vi "crop_input_images.vi"() -> ()   [LabVIEW 2011]
uses:
  global_vars.vi
  <vilib>/Utility/file.llb/Write To Spreadsheet File (I64).vi
  <vilib>/vision/NI_Vision_Development_Module.lvlib
panel:
  in  "Numeric Control":dbl=0.454545454
  out "input_line_plot 2":dbl[][](graph)
  in  "Tab Control":T1(tab)
  out "input_line_plot":u8[][](graph)
  out "img_dist_input":T2(plugin-control)
  out "img_orig_input":T2(plugin-control)
  in  "i32_sel_input_image":i32
  in  "select row input":i32(slide) scale=0.0..1200.0
  in  "select row unwrapped":i32(slide) scale=0.0..1200.0
  out "img_dist_phaseMap":T2(plugin-control)
  out "img_orig_masked_with_dist":T2(plugin-control)
  out "noise_mask_line_plot":u8[](graph)
  out "img_noise_maks":T2(plugin-control)
  out "i32_First/last px":i32[][](graph)
  in  "select row":i32(slide) scale=0.0..1200.0
  out "last px":i32
  out "first px":i32
  in  "save data":bool
  out "i32_ar_displ_map":i32[][](array[numeric])
  in  "safety margin":i32=5
  out "u8_ar_noise_mask":u8[][](array[numeric])
  out "crunching numbers":bool
  out "Intensity Graph":i32[][](graph)
  out "u8_ar_orig_phase_masked_with_dist":u8[][](array[numeric])
  in  "noise threshold":dbl=20.0
  out "img_orig_unwrap":T2(plugin-control)
  in  "calc difference":bool
  out "Y Resolution":i32
  out "X Resolution":i32
  in  "update_cor":bool
  out "path_dist_files":path[](array[path])=[path "X:/Cloud Drives/Dropbox/Europhotonics/FringeMan/Image Storage/02_07/x-direction/dist/12_56_10-5.00fringes_0of4__capt_.png", path "X:/Cloud Drives/Dropbox/Europhotonics/FringeMan/Image Storage/02_07/x-direction/dist/12_56_10-5.00fringes_1of4__capt_.png", path "X:/Cloud Drives/Dropbox/Europhotonics/FringeMan/Image Storage/02_07/x-direction/dist/12_56_10-5.00fringes_2of4__capt_.png", path "X:/Cloud Drives/Dropbox/Europhotonics/FringeMan/Image Storage/02_07/x-direction/dist/12_56_10-5.00fringes_3of4__capt_.png"]
  out "path_orig_files":path[](array[path])=[path "X:/Cloud Drives/Dropbox/Europhotonics/FringeMan/Image Storage/02_07/x-direction/orig/12_56_10-5.00fringes_0of4__original_.png", path "X:/Cloud Drives/Dropbox/Europhotonics/FringeMan/Image Storage/02_07/x-direction/orig/12_56_10-5.00fringes_1of4__original_.png", path "X:/Cloud Drives/Dropbox/Europhotonics/FringeMan/Image Storage/02_07/x-direction/orig/12_56_10-5.00fringes_2of4__original_.png", path "X:/Cloud Drives/Dropbox/Europhotonics/FringeMan/Image Storage/02_07/x-direction/orig/12_56_10-5.00fringes_3of4__original_.png"]
  in  "dbl_ar_crop_correction":dbl[](array[numeric])=[0.0, 0.0, 0.0, 0.0] caption="crop_correction"
  in  "u8_y_center_cor":i16
  in  "u8_x_center_cor":i16=-20
  in  "radius correction":i16=-30
  out "img_dist_unwrap":T2(plugin-control)
  out "u8_ar_orig_phasemap":u8[][](array[numeric])
  out "dbl_pxar_orig_unwrap":u8[][](array[numeric])
  out "dbl_pxar_dist_unwrap":u8[][](array[numeric])
  out "u8_pxar_orig":u8[][][](array[numeric])
  in  "read orig":bool
  in  "read dist":bool
  out "u8_ar_dist_phasemap":u8[][](array[numeric])
  in  "calculate \nphase map":bool
  out "u8_pxar_dist":u8[][][](array[numeric])
  in  "Stop Button":bool
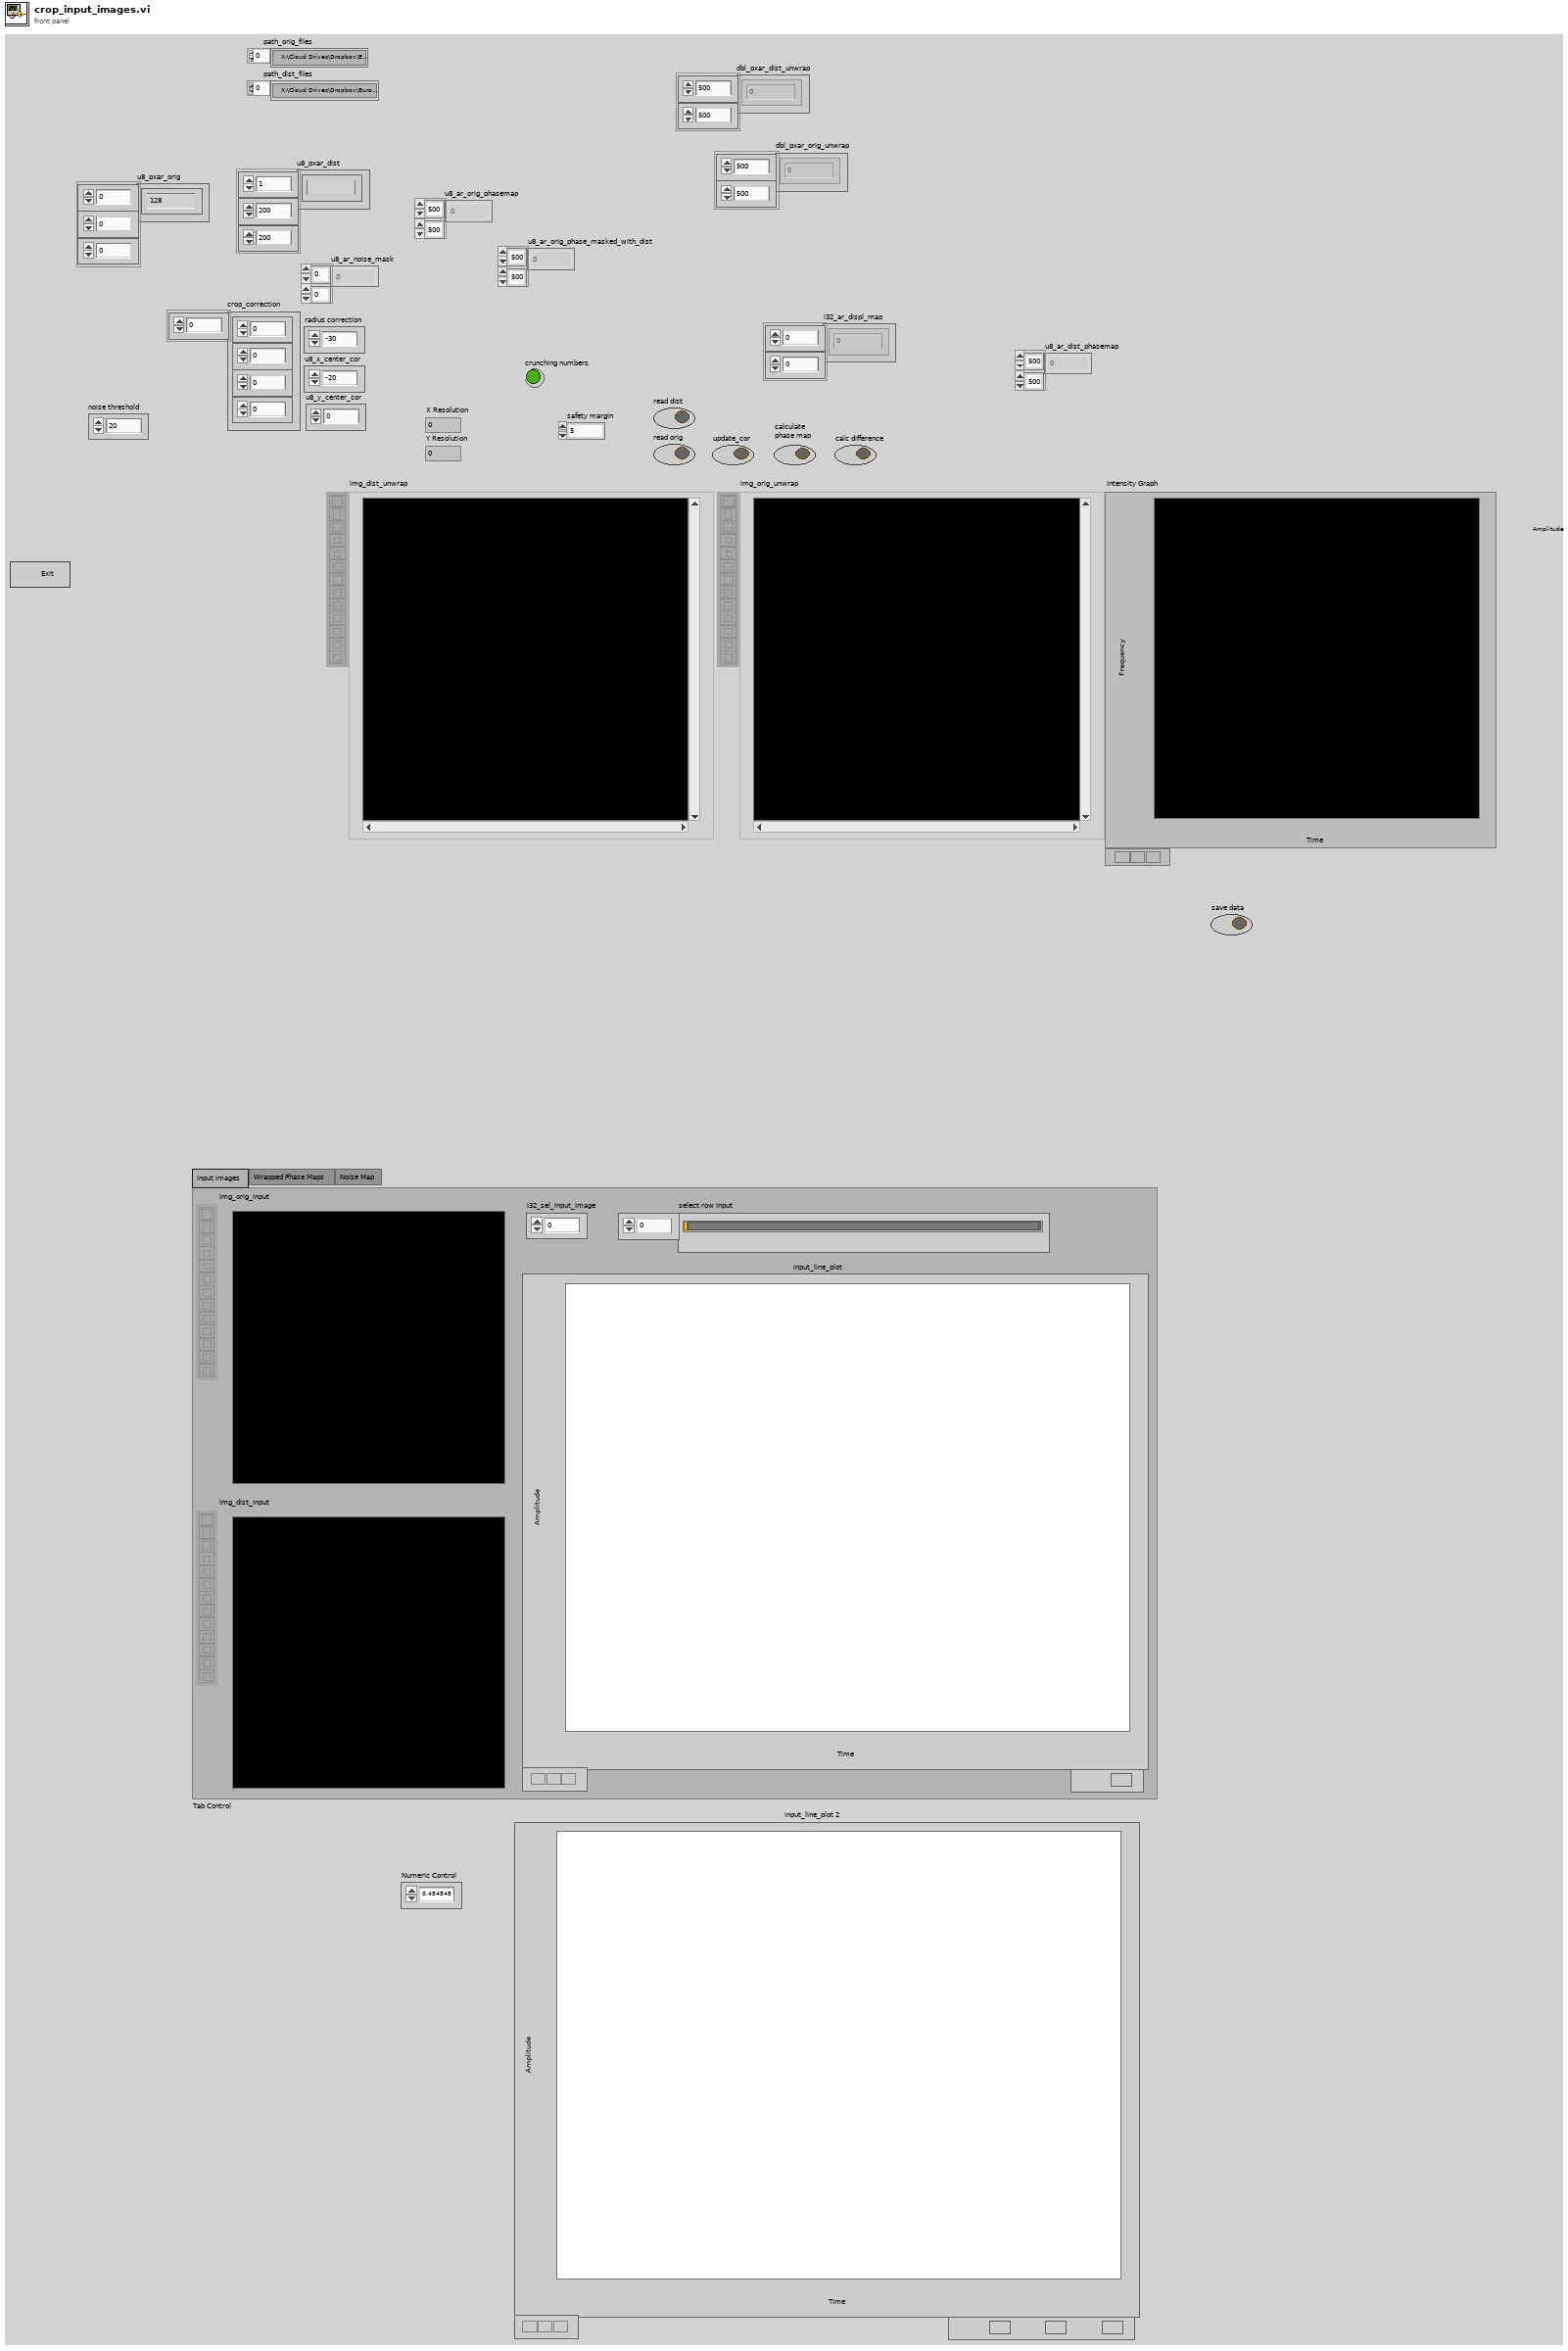
[diagram p1: front panel]
types:
  T1 = enum32{"Input Images", "Wrapped Phase Maps", "Noise Map"}
  T2 = typedef "IMAQ Image.ctl" = refnum<image>
  T3 = typedef "Image Type" = u32
  T4 = cluster{"radius correction":i16, "u8_x_center_cor":i16, "u8_y_center_cor":i16}
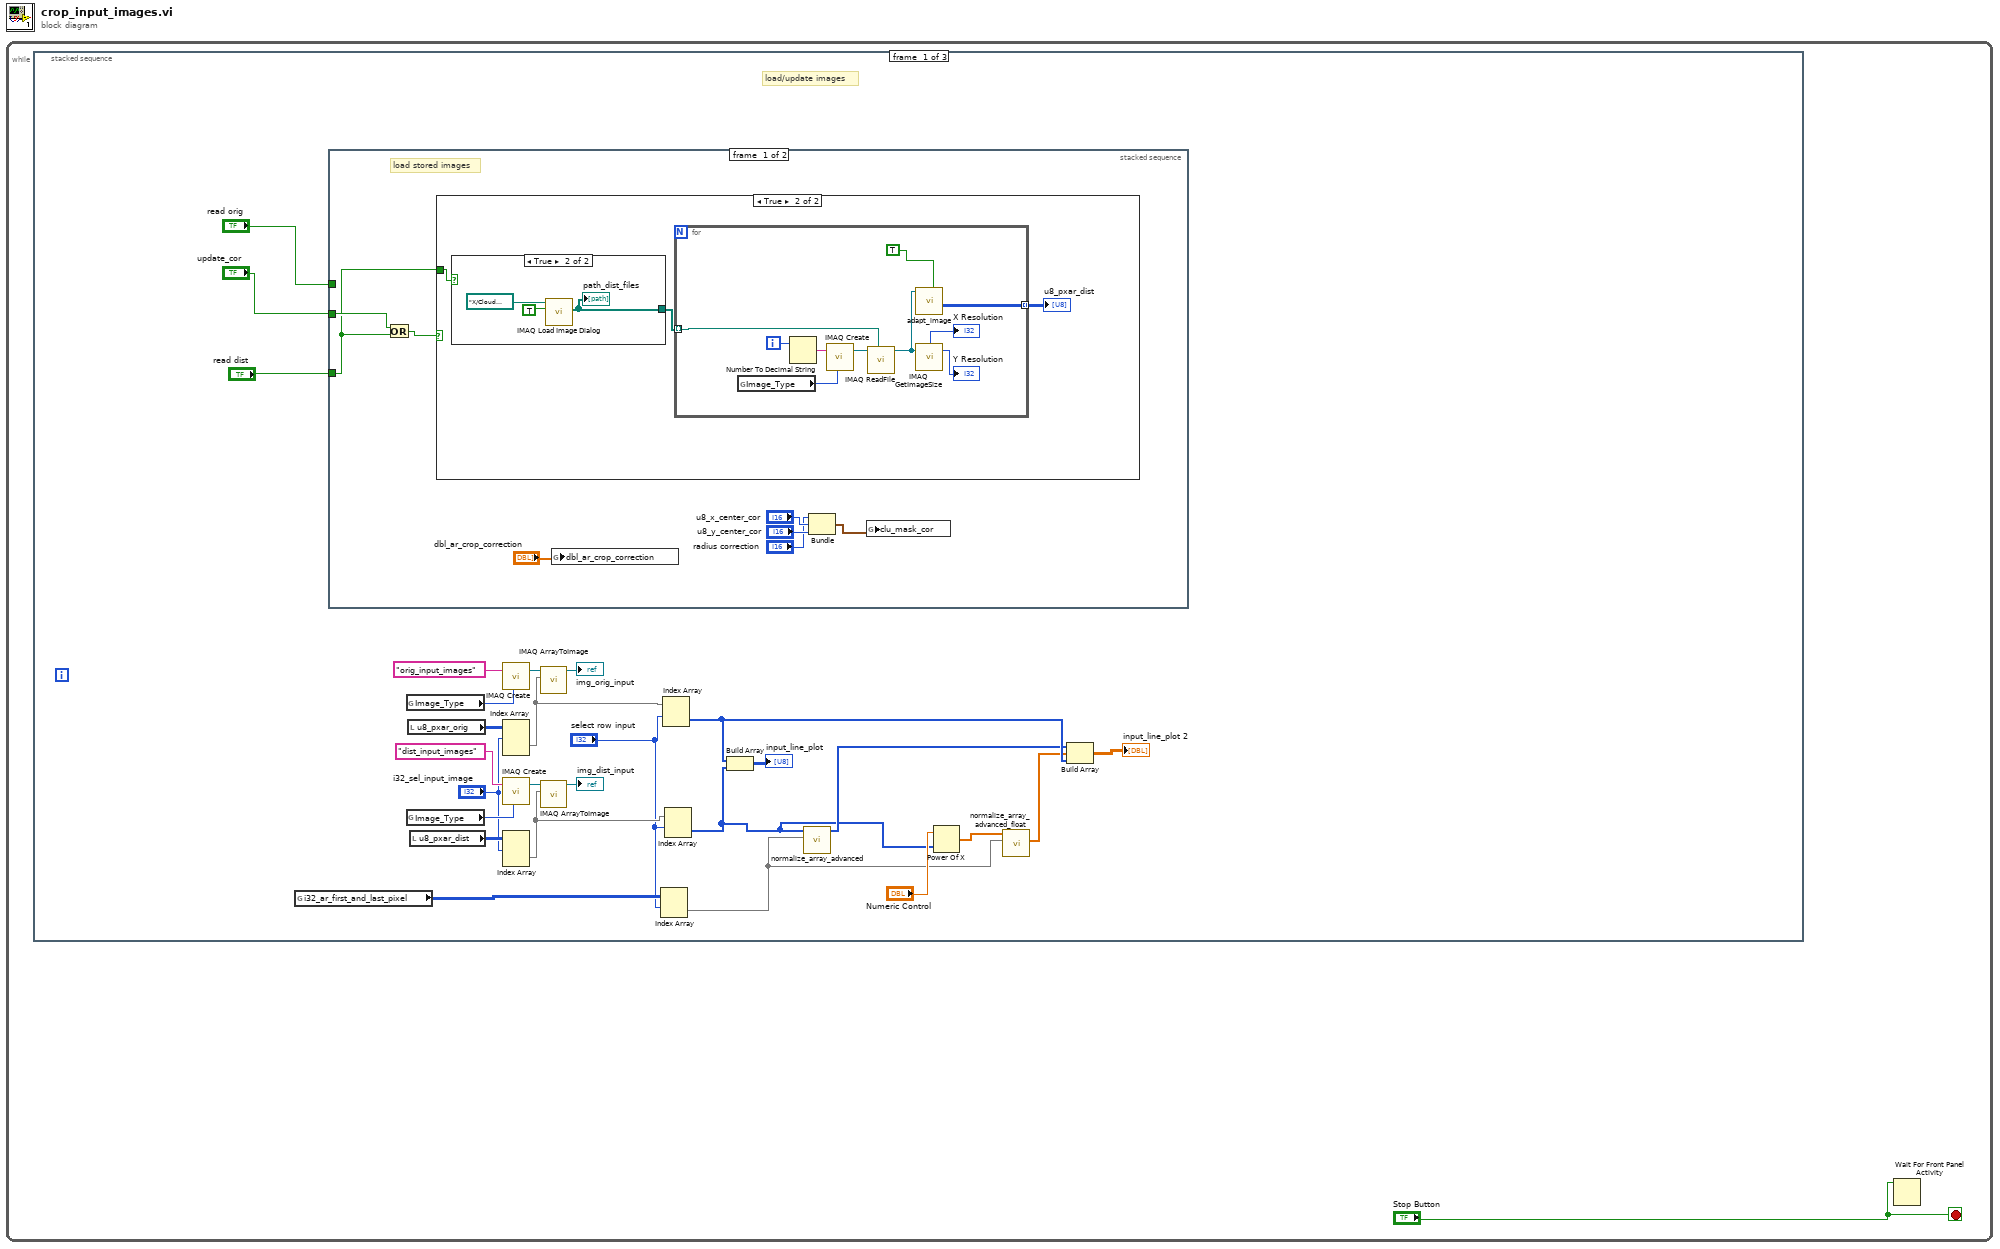
[diagram p0: block diagram]
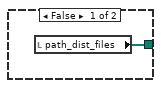
[diagram p3: hidden frame]
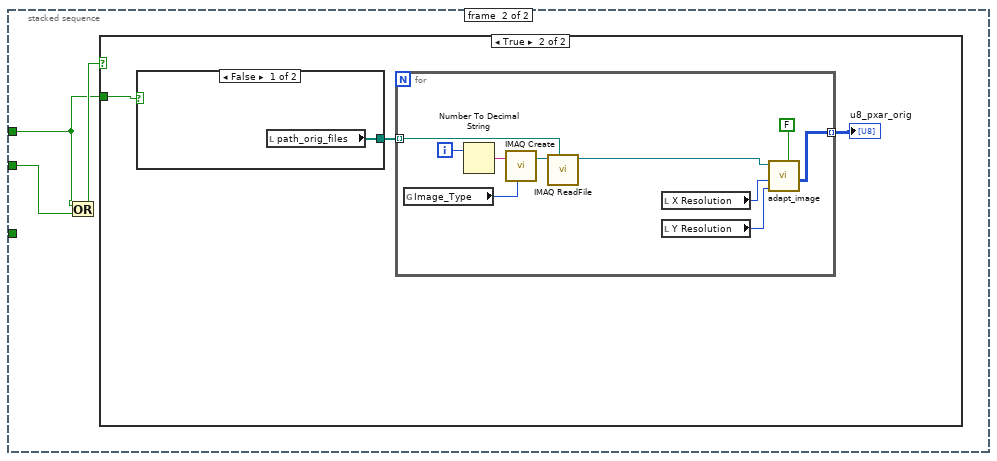
[diagram p4: hidden frame]
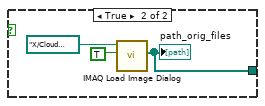
[diagram p6: hidden frame]
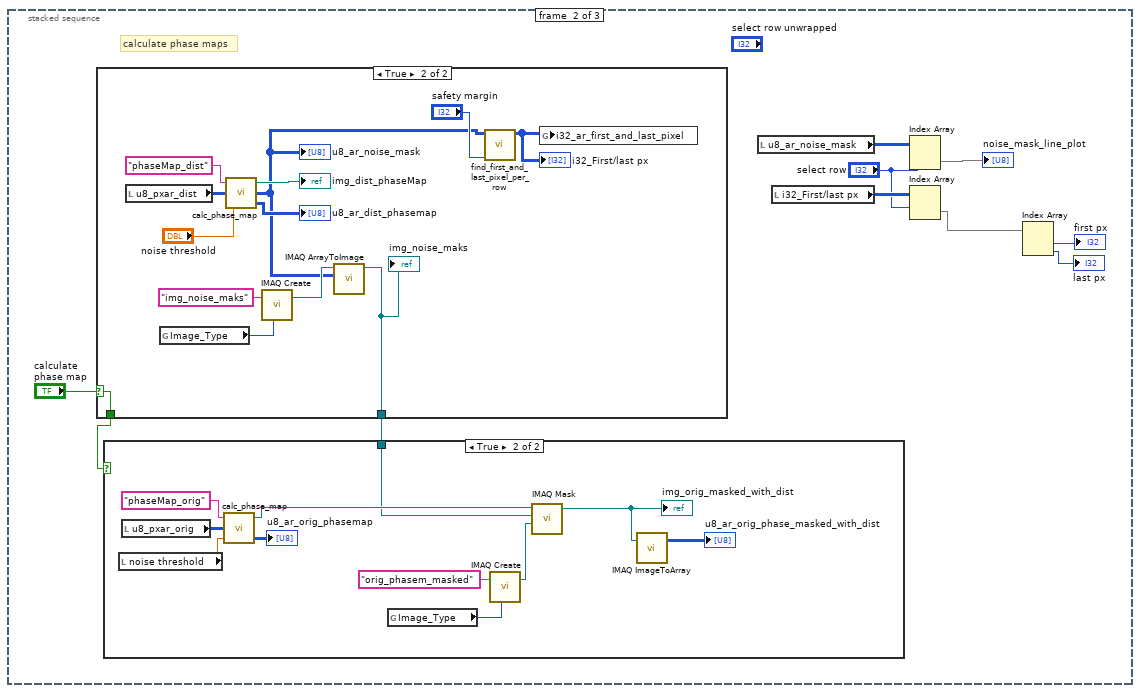
[diagram p7: hidden frame]
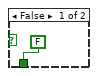
[diagram p9: hidden frame]
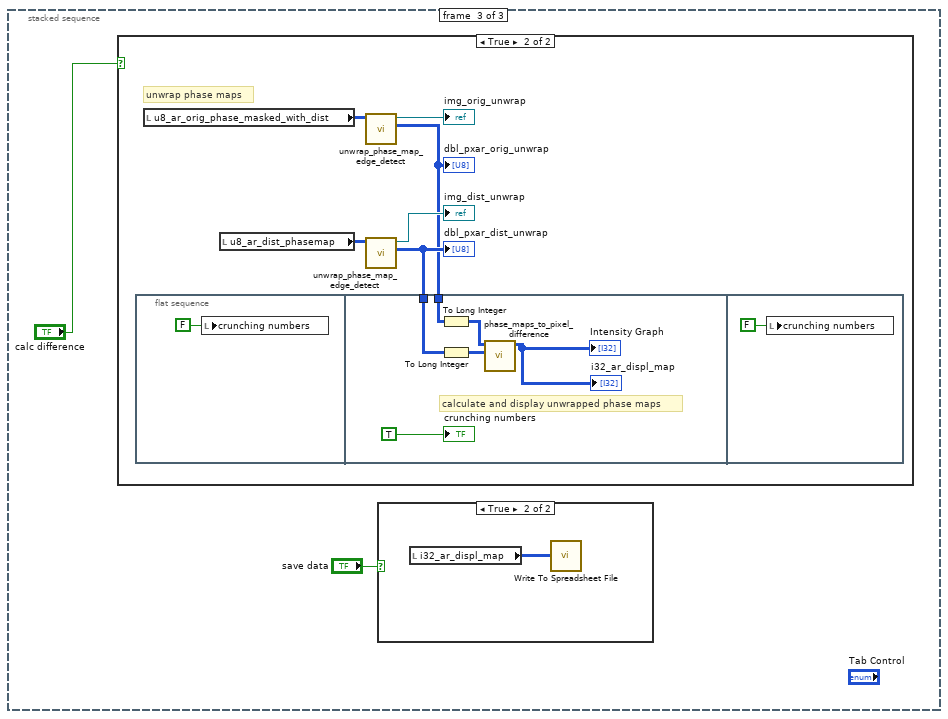
[diagram p10: hidden frame]
diagram:
  n1 = while {
    stop <- "Stop Button" stop-if-true
    n2 = stacked-sequence {
      frame #0 {
        # "load/update images"
        n3 = global read "global_vars.vi" "i32_ar_first_and_last_pixel"() -> (w10:i32[][])
        n4 = stacked-sequence {
          tunnel: "update_cor" -> [w36 w55]
          tunnel: "read dist" -> [w34 _]
          tunnel: "read orig" -> [_ w54]
          frame #0 {
            # "load stored images"
            n5 = Or(x=w36, y=w34) -> (x .or. y?=w35:bool)
            n6 = case shown="True" w35 {
              tunnel: w34 -> [_ w37]
              frame False {
              }
              frame True {
                n7 = case shown="True" w37 {
                  tunnel: [w40 w43] -> w39
                  frame False {
                    n8 = local read "path_dist_files"() -> (w40:path[])
                  }
                  frame True {
                    n9 = call "IMAQ Load Image Dialog"("Multiple Files? (No)"=TRUE, "Start Path"=path "X:/Cloud Drives/Dropbox/Europhotonics/FringeMan/Image Storage") -> ("Paths"=w43:path[])  [unwired: 7 in, 2 out]
                    "path_dist_files" <- w43
                  }
                }
                n10 = for {
                  tunnel: w39 -> [w49] mode=indexing
                  tunnel: [w45] -> w38 mode=indexing
                  i -> [w53]
                  n11 = global read "global_vars.vi" "Image_Type"() -> (w50:T3)
                  n12 = Number To Decimal String(number=w53) -> (decimal integer string=w52:string)  [unwired: 1 in]
                  n13 = call "IMAQ Create"("Image Name"=w52, "Image Type"=w50) -> ("New Image"=w51:T2)  [unwired: 2 in, 2 out]
                  n14 = call "IMAQ ReadFile"("File Path"=w49, "Image"=w51) -> ("Image Out"=w46:T2)  [unwired: 5 in, 4 out]
                  n15 = call "adapt_image.vi"("captured image?"=TRUE, "orig_imageIn"=w46) -> ("adapted image px array"=w45:u8[][])  [unwired: 7 in, 2 out]
                  n16 = call "IMAQ GetImageSize"("Image"=w46) -> ("Y Resolution"=→"Y Resolution":i32, "X Resolution"=→"X Resolution":i32)  [unwired: 3 in, 1 out]
                }
                "u8_pxar_dist" <- w38
              }
            }
            n17 = global write "global_vars.vi" "dbl_ar_crop_correction"("dbl_ar_crop_correction") -> ()
            n18 = Bundle("radius correction"="radius correction", "u8_x_center_cor"="u8_x_center_cor", "u8_y_center_cor"="u8_y_center_cor") -> (w33:T4)  [unwired: 1 in]
            n19 = global write "global_vars.vi" "clu_mask_cor"(w33) -> ()
          }
          frame #1 {
            n20 = Or(x=w54, y=w55) -> (x .or. y?=w56:bool)
            n21 = case shown="True" w56 {
              tunnel: w54 -> [_ w57]
              frame False {
              }
              frame True {
                n22 = case shown="False" w57 {
                  tunnel: [w60 w62] -> w58
                  frame False {
                    n23 = local read "path_orig_files"() -> (w60:path[])
                  }
                  frame True {
                    n24 = call "IMAQ Load Image Dialog"("Multiple Files? (No)"=TRUE, "Start Path"=path "X:/Cloud Drives/Dropbox/Europhotonics/FringeMan/Image Storage") -> ("Paths"=w62:path[])  [unwired: 7 in, 2 out]
                    "path_orig_files" <- w62
                  }
                }
                n25 = for {
                  tunnel: w58 -> [w73] mode=indexing
                  tunnel: [w65] -> w59 mode=indexing
                  i -> [w69]
                  n26 = global read "global_vars.vi" "Image_Type"() -> (w70:T3)
                  n27 = Number To Decimal String(number=w69) -> (decimal integer string=w72:string)  [unwired: 1 in]
                  n28 = call "IMAQ Create"("Image Name"=w72, "Image Type"=w70) -> ("New Image"=w71:T2)  [unwired: 2 in, 2 out]
                  n29 = call "IMAQ ReadFile"("File Path"=w73, "Image"=w71) -> ("Image Out"=w68:T2)  [unwired: 5 in, 4 out]
                  n30 = local read "X Resolution"() -> (w67:i32)
                  n31 = local read "Y Resolution"() -> (w66:i32)
                  n32 = call "adapt_image.vi"("captured image?"=FALSE, "captImage_Y_Resolution"=w66, "captImage_X_Resolution"=w67, "orig_imageIn"=w68) -> ("adapted image px array"=w65:u8[][])  [unwired: 5 in, 2 out]
                }
                "u8_pxar_orig" <- w59
              }
            }
          }
        }
        n33 = global read "global_vars.vi" "Image_Type"() -> (w23:T3)
        n34 = global read "global_vars.vi" "Image_Type"() -> (w20:T3)
        n35 = local read "u8_pxar_orig"() -> (w24:u8[][][])
        n36 = local read "u8_pxar_dist"() -> (w25:u8[][][])
        n37 = call "IMAQ Create"("Image Name"="orig_input_images", "Image Type"=w23) -> ("New Image"=w18:T2)  [unwired: 2 in, 2 out]
        n38 = Index Array(array=w24, index (dim 0)="i32_sel_input_image") -> (element=w15:u8[][])  [unwired: 2 in]
        n39 = call "IMAQ Create"("Image Name"="dist_input_images", "Image Type"=w20) -> ("New Image"=w19:T2)  [unwired: 2 in, 2 out]
        n40 = Index Array(array=w25, index (dim 0)="i32_sel_input_image") -> (element=w14:u8[][])  [unwired: 2 in]
        n41 = call "IMAQ ArrayToImage"("Image Pixels (U8)"=w15, "Image"=w18) -> ("Image Out"=→"img_orig_input":T2)  [unwired: 8 in, 1 out]
        n42 = call "IMAQ ArrayToImage"("Image Pixels (U8)"=w14, "Image"=w19) -> ("Image Out"=→"img_dist_input":T2)  [unwired: 8 in, 1 out]
        n43 = Index Array(array=w10, index (row)="select row input") -> (element=w5:i32[])  [unwired: 1 in]
        n44 = Index Array(array=w15, index (row)="select row input") -> (element=w12:u8[])  [unwired: 1 in]
        n45 = Index Array(array=w14, index (row)="select row input") -> (element=w3:u8[])  [unwired: 1 in]
        n46 = Build Array(w12, w3) -> (→"input_line_plot":u8[][])
        n47 = call "normalize_array_advanced.vi"("i32_ar_first_and_last_pixel"=w5, "unwrapped array"=w3) -> ("normalized unwrapped array"=w8:u8[])  [unwired: 5 in, 4 out]
        n48 = Power Of X(1:w3, 2:"Numeric Control") -> (0:w2:dbl[])
        n49 = call "normalize_array_advanced_float.vi"("i32_ar_first_and_last_pixel"=w5, "unwrapped array"=w2) -> ("i16_normalized unwrapped array"=w4:dbl[])  [unwired: 5 in, 4 out]
        n50 = Build Array(w8, w4, w12) -> (→"input_line_plot 2":dbl[][])
      }
      frame #1 {
        # "calculate phase maps"
        n51 = case shown="True" "calculate \nphase map" {
          selector: "calculate \nphase map" -> [_ w106]
          tunnel: [FALSE w106] -> w82
          tunnel: [_ w98] -> w81
          frame False {
          }
          frame True {
            n52 = local read "u8_pxar_dist"() -> (w107:u8[][][])
            n53 = global read "global_vars.vi" "Image_Type"() -> (w101:T3)
            n54 = call "calc_phase_map.vi"("noise threshold"="noise threshold", "u8_ar_image_pixel_array"=w107, "image name"="phaseMap_dist" ("String")) -> ("raw phase map array"=→"u8_ar_dist_phasemap":u8[][], "u8_ar_noise_mask"=w96:u8[][], "phase map"=→"img_dist_phaseMap":T2)
            "u8_ar_noise_mask" <- w96
            n55 = call "IMAQ Create"("Image Name"="img_noise_maks", "Image Type"=w101) -> ("New Image"=w100:T2)  [unwired: 2 in, 2 out]
            n56 = call "IMAQ ArrayToImage"("Image Pixels (U8)"=w96, "Image"=w100) -> ("Image Out"=w98:T2)  [unwired: 8 in, 1 out]
            "img_noise_maks" <- w98
            n57 = call "find_first_and_last_pixel_per_row.vi"("safety margin"="safety margin", "u8_ar_mask"=w96) -> ("i32_ar_first_and_last_pixel"=w97:i32[][])  [unwired: 9 in]
            "i32_First/last px" <- w97
            n58 = global write "global_vars.vi" "i32_ar_first_and_last_pixel"(w97) -> ()
          }
        }
        n59 = case shown="True" w82 {
          tunnel: w81 -> [_ w84]
          frame False {
          }
          frame True {
            n60 = local read "noise threshold"() -> (w91:dbl)
            n61 = local read "u8_pxar_orig"() -> (w93:u8[][][])
            n62 = call "calc_phase_map.vi"("noise threshold"=w91, "u8_ar_image_pixel_array"=w93, "image name"="phaseMap_orig" ("String")) -> ("raw phase map array"=→"u8_ar_orig_phasemap":u8[][], "phase map"=w90:T2)  [unwired: 1 out]
            n63 = global read "global_vars.vi" "Image_Type"() -> (w89:T3)
            n64 = call "IMAQ Create"("Image Name"="orig_phasem_masked", "Image Type"=w89) -> ("New Image"=w88:T2)  [unwired: 2 in, 2 out]
            n65 = call "IMAQ Mask"("Image Dst"=w88, "Image Mask"=w84, "Image Src"=w90) -> ("Image Dst Out"=w86:T2)  [unwired: 2 in, 1 out]
            "img_orig_masked_with_dist" <- w86
            n66 = call "IMAQ ImageToArray"("Image"=w86) -> ("Image Pixels (U8)"=→"u8_ar_orig_phase_masked_with_dist":u8[][])  [unwired: 3 in, 4 out]
          }
        }
        n67 = local read "u8_ar_noise_mask"() -> (w80:u8[][])
        n68 = local read "i32_First/last px"() -> (w79:i32[][])
        n69 = Index Array(array=w80, index (row)="select row") -> (element=→"noise_mask_line_plot":u8[])  [unwired: 1 in]
        n70 = Index Array(array=w79, index (row)="select row") -> (element=w76:i32[])  [unwired: 1 in]
        n71 = Index Array(array=w76) -> (element #1=→"first px":i32, element #2=→"last px":i32)  [unwired: 2 in]
      }
      frame #2 {
        n72 = case shown="True" "calc difference" {
          frame False {
          }
          frame True {
            # "unwrap phase maps"
            n73 = flat-sequence {
              tunnel: w113 -> [w123]
              tunnel: w112 -> [w122]
              frame #0 {
                n74 = local write "crunching numbers"(FALSE) -> ()
              }
              frame #1 {
                # "calculate and display unwrapped phase maps"
                n75 = To Long Integer(number=w122) -> (32bit integer=w121:i32[][])
                n76 = To Long Integer(number=w123) -> (32bit integer=w120:i32[][])
                n77 = call "phase_maps_to_pixel_difference.vi"("dist phase map"=w120, "oirg phase map"=w121) -> ("displacement map"=→"Intensity Graph" →"i32_ar_displ_map":i32[][])  [unwired: 9 in]
                "crunching numbers" <- TRUE
              }
              frame #2 {
                n78 = local write "crunching numbers"(FALSE) -> ()
              }
            }
            n79 = local read "u8_ar_orig_phase_masked_with_dist"() -> (w114:u8[][])
            n80 = local read "u8_ar_dist_phasemap"() -> (w115:u8[][])
            n81 = call "unwrap_phase_map_edge_detect.vi"("u8_ar_dist_phasemap"=w114) -> ("df_ar_unwrapped_px_ar"=w112:u8[][], "Refnum out"=→"img_orig_unwrap":T2)  [unwired: 9 in]
            "dbl_pxar_orig_unwrap" <- w112
            n82 = call "unwrap_phase_map_edge_detect.vi"("u8_ar_dist_phasemap"=w115) -> ("df_ar_unwrapped_px_ar"=w113:u8[][], "Refnum out"=→"img_dist_unwrap":T2)  [unwired: 9 in]
            "dbl_pxar_dist_unwrap" <- w113
          }
        }
        n83 = case shown="True" "save data" {
          frame False {
          }
          frame True {
            n84 = local read "i32_ar_displ_map"() -> (w111:i32[][])
            n85 = call-poly <vilib>:"Write To Spreadsheet File.vi"("2D data"=w111) -> ()  [unwired: 7 in, 1 out]
          }
        }
      }
    }
    n86 = Wait For Front Panel Activity(3:"Stop Button") -> ()  [unwired: 2 in, 1 out]
  }
